vi "DataTreeCtrl init.vi"(8 "error in (no error)":errorcluster, 11 "DataTreeCtrl in":refnum<class "DataTreeCtrl.lvclass">) -> (0 "error out":errorcluster, 3 "DataTreeCtrl out":refnum<class "DataTreeCtrl.lvclass">)   [LabVIEW 2018, in "DataTreeCtrl.lvclass"]
uses:
  DataTreeCtrl.lvclass
  ctl/FMstateMachineEnum.ctl
  DataTreeCtrl.lvclass/DataTreeCtrl.ctl
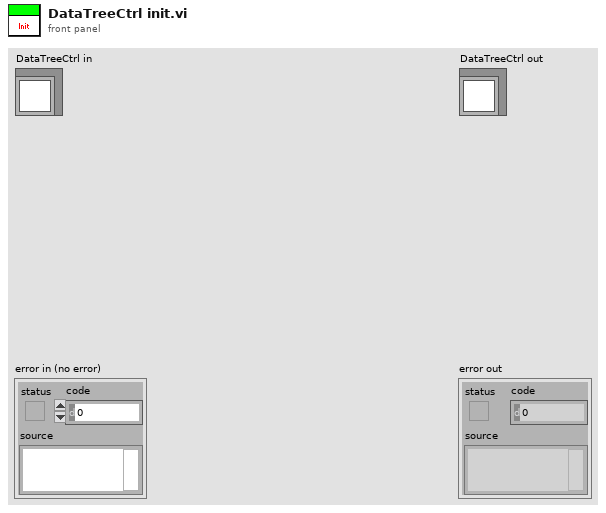
[diagram p1: front panel]
types:
  T1 = typedef "FMstateMachineEnum.ctl" = enum16{"none", "init", "openTDMS", "closeTDMS", "getDataList", "getDataInfo", "getTimeStamp", "getCurrPath", "getRemark", "overwriteRemark", "readData", "deleteData", "moveData"}
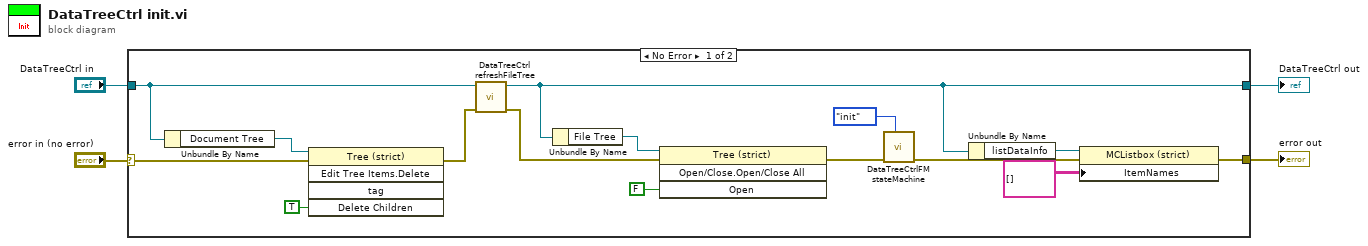
[diagram p0: block diagram]
diagram:
  n1 = case shown="No Error" "error in (no error)" {
    selector: "error in (no error)" -> [w17 w21]
    tunnel: [w5 w21] -> w3
    tunnel: [w9 w20] -> w1
    tunnel: "DataTreeCtrl in" -> [w16 w20]
    frame No Error {
      n2 = Unbundle By Name(w16) -> ("Document Tree"=w19:refnum<vi>)
      n3 = invoke class="Tree (strict)" method="Edit Tree Items.Delete"(reference=w19, error in=w17, "Delete Children"=TRUE ("Delete Children?")) -> (error out=w15:errorcluster)  [unwired: 2 in, 4 out]
      n4 = call "DataTreeCtrl refreshFileTree.vi"("error in (no error)"=w15, "DataTreeCtrl in"=w16) -> ("error out"=w13:errorcluster, "DataTreeCtrl out"=w9:refnum<class "DataTreeCtrl.lvclass">)  [unwired: 8 in]
      n5 = Unbundle By Name(w9) -> ("File Tree"=w12:refnum<vi>)
      n6 = invoke class="Tree (strict)" method="Open/Close.Open/Close All"(reference=w12, error in=w13, "Open"=FALSE ("Open?")) -> (error out=w10:errorcluster)  [unwired: 1 in, 3 out]
      n7 = call "DataTreeCtrlFM stateMachine.vi"("Func"=FMstateMachineEnum."init", "error in (no error)"=w10) -> ("error out"=w7:errorcluster)  [unwired: 4 in, 5 out]
      n8 = Unbundle By Name(w9) -> ("listDataInfo"=w8:refnum<vi>)
      n9 = property class="MCListbox (strict)"(reference=w8, error in=w7, "ItemNames"=string[][] [] ("Item Names")) -> (error out=w5:errorcluster)  [unwired: 1 out]
    }
    frame Error {
    }
  }
  "error out" <- w3
  "DataTreeCtrl out" <- w1
